vi "Update.vi"(8 "error in (no error)":errorcluster, 11 "Snake in":refnum<class "SnakeGame.lvclass">) -> (0 "error out":errorcluster, 3 "Snake out":refnum<class "SnakeGame.lvclass">)   [LabVIEW 2019, in "RT_Game.lvlib" / "SnakeGame.lvclass"]
uses:
  SnakeGame.lvclass
  C:/Users/FreshBob/Dropbox/VIs/myRIO_GameConsole/RT/RT_Game/Game/Game.lvclass
  SnakeGame.lvclass/SnakeGame.ctl
  Snake/Snake.lvclass/Snake.ctl
  Game/Game.lvclass/Game.ctl
  Snake/Read Dead_.vi
  Write SinglePlayer.vi
  Game/Write FlattenedNextClass.vi
  Game/Game.lvclass
  Snake/Snake.lvclass
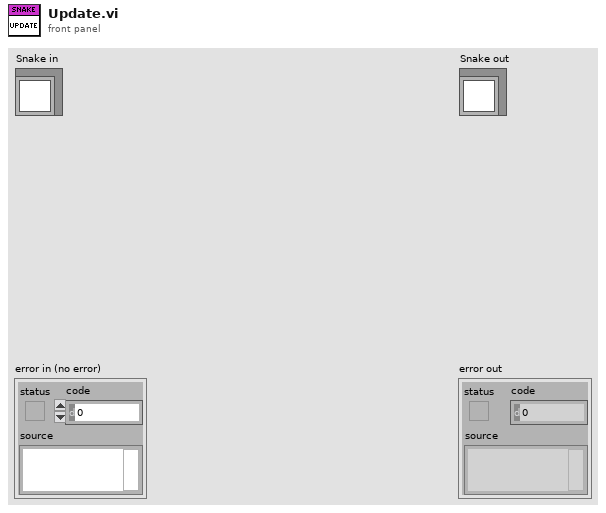
[diagram p1: front panel]
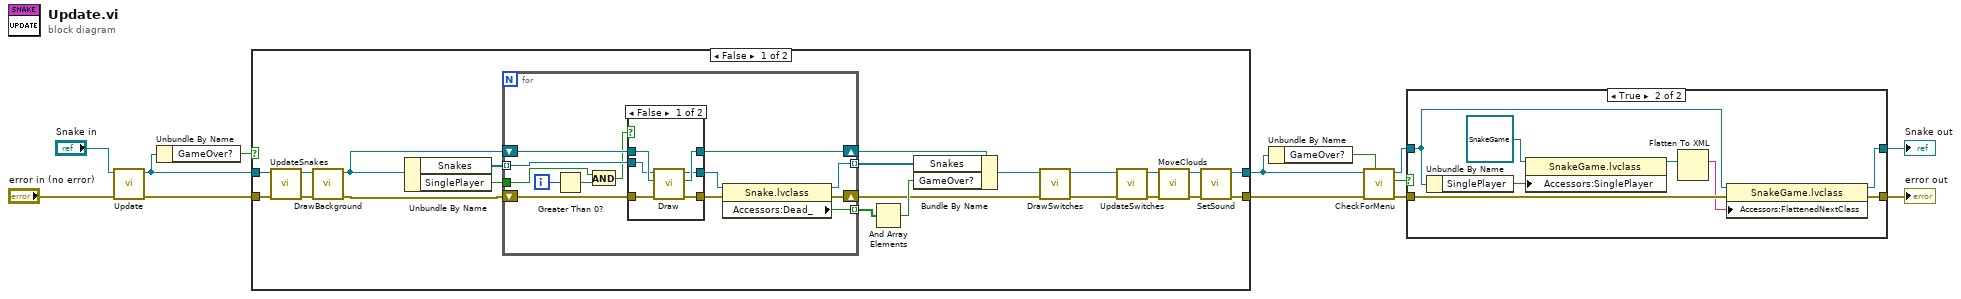
[diagram p0: block diagram]
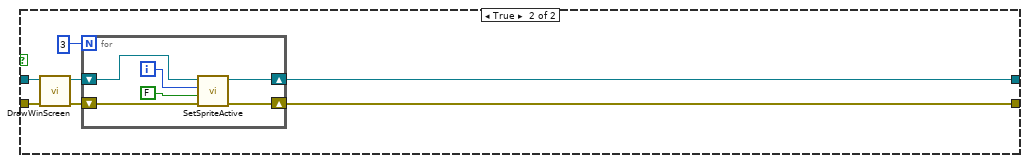
[diagram p4: hidden frame]
diagram:
  n1 = call-parent "Update.vi"("error in (no error)"="error in (no error)", "Game in"="Snake in") -> ("error out"=w13:errorcluster, "Game out"=w8:refnum<class "SnakeGame.lvclass">)  [unwired: 8 in]
  n2 = Unbundle By Name(w8) -> ("GameOver?"=w7:bool)
  n3 = case shown="False" w7 {
    tunnel: w13 -> [w17 w63]
    tunnel: [w26 w62] -> w6
    tunnel: [w28 w61] -> w9
    tunnel: w8 -> [w18 w59]
    frame False {
      n4 = call "UpdateSnakes.vi"("error in (no error)"=w17, "SnakeGame in"=w18) -> ("error out"=w24:errorcluster, "SnakeGame out"=w25:refnum<class "SnakeGame.lvclass">)  [unwired: 8 in]
      n5 = call "DrawBackground.vi"("error in (no error)"=w24, "Snake in"=w25) -> ("error out"=w23:errorcluster, "Snake out"=w22:refnum<class "SnakeGame.lvclass">)  [unwired: 8 in]
      n6 = Unbundle By Name(w22) -> ("Snakes"=w33:refnum<class "Snake.lvclass">[], "SinglePlayer"=w29:bool)
      n7 = for {
        tunnel: w33 -> [w47] mode=indexing
        tunnel: [w41] -> w32 mode=indexing
        shift-right: [w43] -> w19
        shift-left: w23 -> [w48]
        shift-right: [w44] -> w34
        shift-left: w22 -> [w45]
        tunnel: [w40] -> w31 mode=indexing
        tunnel: w29 -> [w37]
        i -> [w39]
        n8 = Greater Than 0?(x=w39) -> (x > 0?=w36:bool)
        n9 = And(x=w37, y=w36) -> (x .and. y?=w38:bool)
        n10 = case shown="False" w38 {
          tunnel: w48 -> [w49 w55]
          tunnel: w47 -> [w50 w56]
          tunnel: [w54 w55] -> w46
          tunnel: w45 -> [w53 w57]
          tunnel: [w52 w57] -> w44
          tunnel: [w51 w56] -> w42
          frame False {
            n11 = call "Draw.vi"("error in (no error)"=w49, "Snake in 2"=w53, "Snake in"=w50) -> ("error out"=w54:errorcluster, "Snake out 2"=w52:refnum<class "SnakeGame.lvclass">, "Snake out"=w51:refnum<class "Snake.lvclass">)  [unwired: 6 in]
          }
          frame True {
          }
        }
        n12 = property class="Snake.lvclass"(reference=w42, error in=w46) -> (reference out=w41:refnum<class "Snake.lvclass">, error out=w43:errorcluster, "Accessors:Dead_"=w40:bool)
      }
      n13 = And Array Elements(Boolean array=w31) -> (logical AND=w30:bool)
      n14 = Bundle By Name(cluster=w34, "Snakes"=w32, "GameOver?"=w30) -> (w15:refnum<class "SnakeGame.lvclass">)
      n15 = call "DrawSwitches.vi"("error in (no error)"=w19, "SnakeGame in"=w15) -> ("error out"=w16:errorcluster, "SnakeGame out"=w14:refnum<class "SnakeGame.lvclass">)  [unwired: 8 in]
      n16 = call "UpdateSwitches.vi"("error in (no error)"=w16, "SnakeGame in"=w14) -> ("error out"=w20:errorcluster, "SnakeGame out"=w21:refnum<class "SnakeGame.lvclass">)  [unwired: 8 in]
      n17 = call "MoveClouds.vi"("error in (no error)"=w20, "SnakeGame in"=w21) -> ("error out"=w35:errorcluster, "SnakeGame out"=w27:refnum<class "SnakeGame.lvclass">)  [unwired: 8 in]
      n18 = call "SetSound.vi"("error in (no error)"=w35, "SnakeGame in"=w27) -> ("error out"=w28:errorcluster, "SnakeGame out"=w26:refnum<class "SnakeGame.lvclass">)  [unwired: 8 in]
    }
    frame True {
      n19 = call "DrawWinScreen.vi"("error in (no error)"=w63, "Snake in"=w59) -> ("error out"=w60:errorcluster, "Snake out"=w58:refnum<class "SnakeGame.lvclass">)  [unwired: 8 in]
      n20 = for {
        N: 3 -> [_]
        shift-right: [w69] -> w61
        shift-left: w60 -> [w70]
        shift-right: [w67] -> w62
        shift-left: w58 -> [w68]
        i -> [w65]
        n21 = call "SetSpriteActive.vi"("error in (no error)"=w70, "Active"=FALSE, "index"=w65, "Game in"=w68) -> ("error out"=w69:errorcluster, "Game out"=w67:refnum<class "SnakeGame.lvclass">)  [unwired: 6 in]
      }
    }
  }
  n22 = Unbundle By Name(w6) -> ("GameOver?"=w5:bool)
  n23 = call "CheckForMenu.vi"("Restart? (F)"=w5, "error in (no error)"=w9, "Snake in"=w6) -> ("error out"=w10:errorcluster, "Restart out"=w1:bool, "Snake out"=w3:refnum<class "SnakeGame.lvclass">)  [unwired: 6 in]
  n24 = case shown="True" w1 {
    tunnel: w10 -> [w71 w80]
    tunnel: [w71 w79] -> w4
    tunnel: w3 -> [w72 w75]
    tunnel: [w72 w78] -> w2
    frame False {
    }
    frame True {
      n25 = Unbundle By Name(w75) -> ("SinglePlayer"=w74:bool)
      n26 = property class="SnakeGame.lvclass"(reference=refnum<class "SnakeGame.lvclass"> refnum ("RT_Game.lvlib:SnakeGame.lvclass"), "Accessors:SinglePlayer"=w74) -> (reference out=w76:refnum<class "SnakeGame.lvclass">)  [unwired: 1 in, 1 out]
      n27 = Flatten To XML(anything=w76) -> (xml string=w73:string)
      n28 = property class="SnakeGame.lvclass"(reference=w75, error in=w80, "Accessors:FlattenedNextClass"=w73) -> (reference out=w78:refnum<class "SnakeGame.lvclass">, error out=w79:errorcluster)
    }
  }
  "error out" <- w4
  "Snake out" <- w2
